vi "TargetSet.vi"(8 "target aim (goal)":dbl[](array[numeric]), 9 "target set (ball)":dbl[](array[numeric]), 11 "pose":dbl[](array[numeric])) -> (1 "target pose out":dbl[](array[numeric]))   [LabVIEW 2016]
panel:
  in  "radius":dbl=150.0
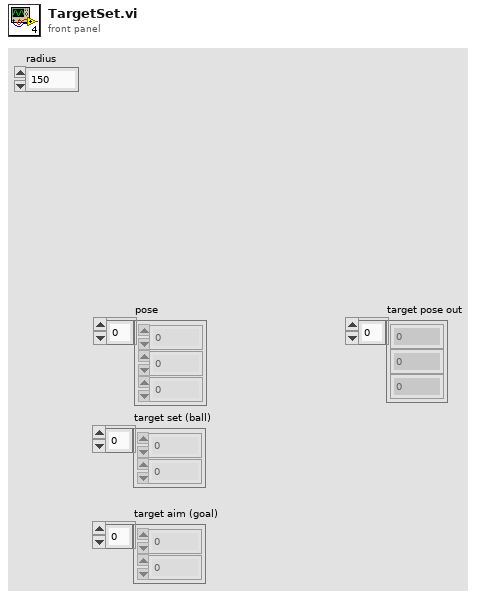
[diagram p1: front panel]
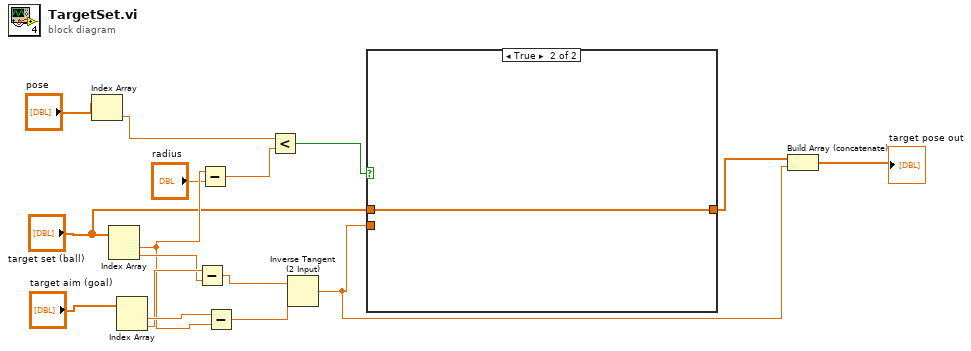
[diagram p0: block diagram]
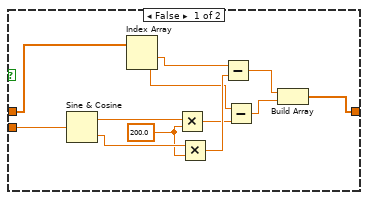
[diagram p2: hidden frame]
diagram:
  n1 = Index Array(array="pose") -> (element=w7:dbl)  [unwired: 1 in]
  n2 = Index Array(array="target set (ball)") -> (element #1=w9:dbl, element #2=w13:dbl)  [unwired: 2 in]
  n3 = Index Array(array="target aim (goal)") -> (element #1=w15:dbl, element #2=w14:dbl)  [unwired: 2 in]
  n4 = Subtract(x=w14, y=w13) -> (x-y=w12:dbl)
  n5 = Subtract(x=w9, y="radius") -> (x-y=w6:dbl)
  n6 = Subtract(x=w15, y=w9) -> (x-y=w11:dbl)
  n7 = Less?(x=w7, y=w6) -> (x < y?=w5:bool)
  n8 = Inverse Tangent (2 Input)(1:w11, 2:w12) -> (0:w2:dbl)
  n9 = case shown="True" w5 {
    tunnel: "target set (ball)" -> [w24 w29]
    tunnel: [w17 w29] -> w3
    tunnel: w2 -> [w28 _]
    frame False {
      w25 = 200.0 ("y")
      n10 = Sine & Cosine(0:w28) -> (1:w27:dbl, 2:w26:dbl)
      n11 = Index Array(array=w24) -> (element #1=w23:dbl, element #2=w21:dbl)  [unwired: 2 in]
      n12 = Multiply(x=w27, y=w25) -> (x*y=w20:dbl)
      n13 = Multiply(x=w26, y=w25) -> (x*y=w22:dbl)
      n14 = Subtract(x=w23, y=w22) -> (x-y=w19:dbl)
      n15 = Subtract(x=w21, y=w20) -> (x-y=w18:dbl)
      n16 = Build Array(w19, w18) -> (w17:dbl[])
    }
    frame True {
    }
  }
  n17 = Build Array (concatenate)(w3, w2) -> (→"target pose out":dbl[])
